vi "Autonomous Independent.vi"   [LabVIEW 2017]
doc: "This VI is called when autonomous begins, and will automatically be terminated when autonomous ends. You can carry out timed or sensor driven robot movement independently without needing to return to the caller."
uses:
  Public/Documents/Cross The Road Electronics/Phoenix-LabVIEW/Motor Controller/Controls/CTRE_Phoenix_MotorControl_ControlMode.ctl
  <vilib>/Rock Robotics/WPI/Utilities/WPI_GetSetVariantRefNum.vi
  <vilib>/Rock Robotics/Network Tables/NT Read String.vi
  <vilib>/Rock Robotics/Network Tables/NT Write Numeric Array.vi
  Public/Documents/Cross The Road Electronics/Phoenix-LabVIEW/Motor Controller/Get/CTRE_Phoenix_MotorController_GetSelectedSensorData.vi
panel:
  # "Be sure to right-click and choose Data Operations>>Make Current Value default if you want to save the array values with the VI"
types:
  T1 = typedef "CTRE_Phoenix_MotorControl_ControlMode.ctl" = u16
  T2 = typedef "WPI_JoystickDevRef.ctl" = cluster{"Device":T3}
  T3 = typedef "WPI_JoystickDeviceEnum.ctl" = enum16{"USB 0", "USB 1", "USB 2", "USB 3", "USB 4", "USB 5"}
  T4 = typedef "WPI_GyroDevRef.ctl" = cluster{"DevStatus":errorcluster, "Analog Channel":T5, "Gain (VoltsPerDegree/Second)":dbl, "Gyro Type":enum16{"Analog", "XRS450"}, "Handle":i32, "SPI Bus":T6, "Device Found":bool, "Sample Rate":dbl, "Calibrate On Open":bool, "Offset":dbl}
  T5 = typedef "FPGA_AIChannel.ctl" = enum8{"AI 0", "AI 1", "AI 2", "AI 3", "AI MXP 0", "AI MXP 1", "AI MXP 2", "AI MXP 3", "Invalid"}
  T6 = typedef "spi_bus.ctl" = enum16{"SPI On-Board, CS0", "SPI On-Board, CS1", "SPI On-Board, CS2", "SPI On-Board, CS3", "SPI MXP", "Invalid"}
  T7 = typedef "WPI_MotorControlDeviceRef.ctl" = cluster{"DeviceStatus":errorcluster, "Type":T8, "PWM":cluster{"PWM Channel":T9, "DeadBand":T10}, "CAN":cluster{"Device Number":u8, "SetOutput VI Ref":variant, "GetOutput VI Ref":variant, "Enable VI Ref":variant, "Disable VI Ref":variant, "Data":variant}, "Invert":bool, "DIO PWM":cluster{"PWM \"Enable\" Channel":T9, "DIOChannel":T11, "PWM Rate":dbl}}
  T8 = typedef "WPI_MotorControlType.ctl" = enum16{"PWM", "CAN", "DIO PWM"}
  T9 = typedef "FPGA_DIOPWMChannel.ctl" = enum8{"PWM 0", "PWM 1", "PWM 2", "PWM 3", "PWM 4", "PWM 5", "PWM 6", "PWM 7", "PWM 8", "PWM 9", "PWM MXP 0", "PWM MXP 1", "PWM MXP 2", "PWM MXP 3", "PWM MXP 4", "PWM MXP 5", "PWM MXP 6", "PWM MXP 7", "PWM MXP 8", "PWM MXP 9", "Invalid"}
  T10 = typedef "WPI_PWMDeadband.ctl" = cluster{"Name":string, "maxPositivePwm":i32, "minPositivePwm":i32, "centerPwm":i32, "maxNegativePwm":i32, "minNegativePwm":i32, "angularRange":u16}
  T11 = typedef "FPGA_DIOChannel.ctl" = enum8{"DIO 0", "DIO 1", "DIO 2", "DIO 3", "DIO 4", "DIO 5", "DIO 6", "DIO 7", "DIO 8", "DIO 9", "DIO MXP 0", "DIO MXP 1", "DIO MXP 2", "DIO MXP 3", "DIO MXP 4", "DIO MXP 5", "DIO MXP 6", "DIO MXP 7", "DIO MXP 8", "DIO MXP 9", "DIO MXP 10", "DIO MXP 11", "DIO MXP 12", "DIO MXP 13", "DIO MXP 14", "DIO MXP 15", "SPI Port CS1", "SPI Port CS2", "SPI Port CS3", "SPI Port MISO", "SPI Port MOSI", "Invalid"}
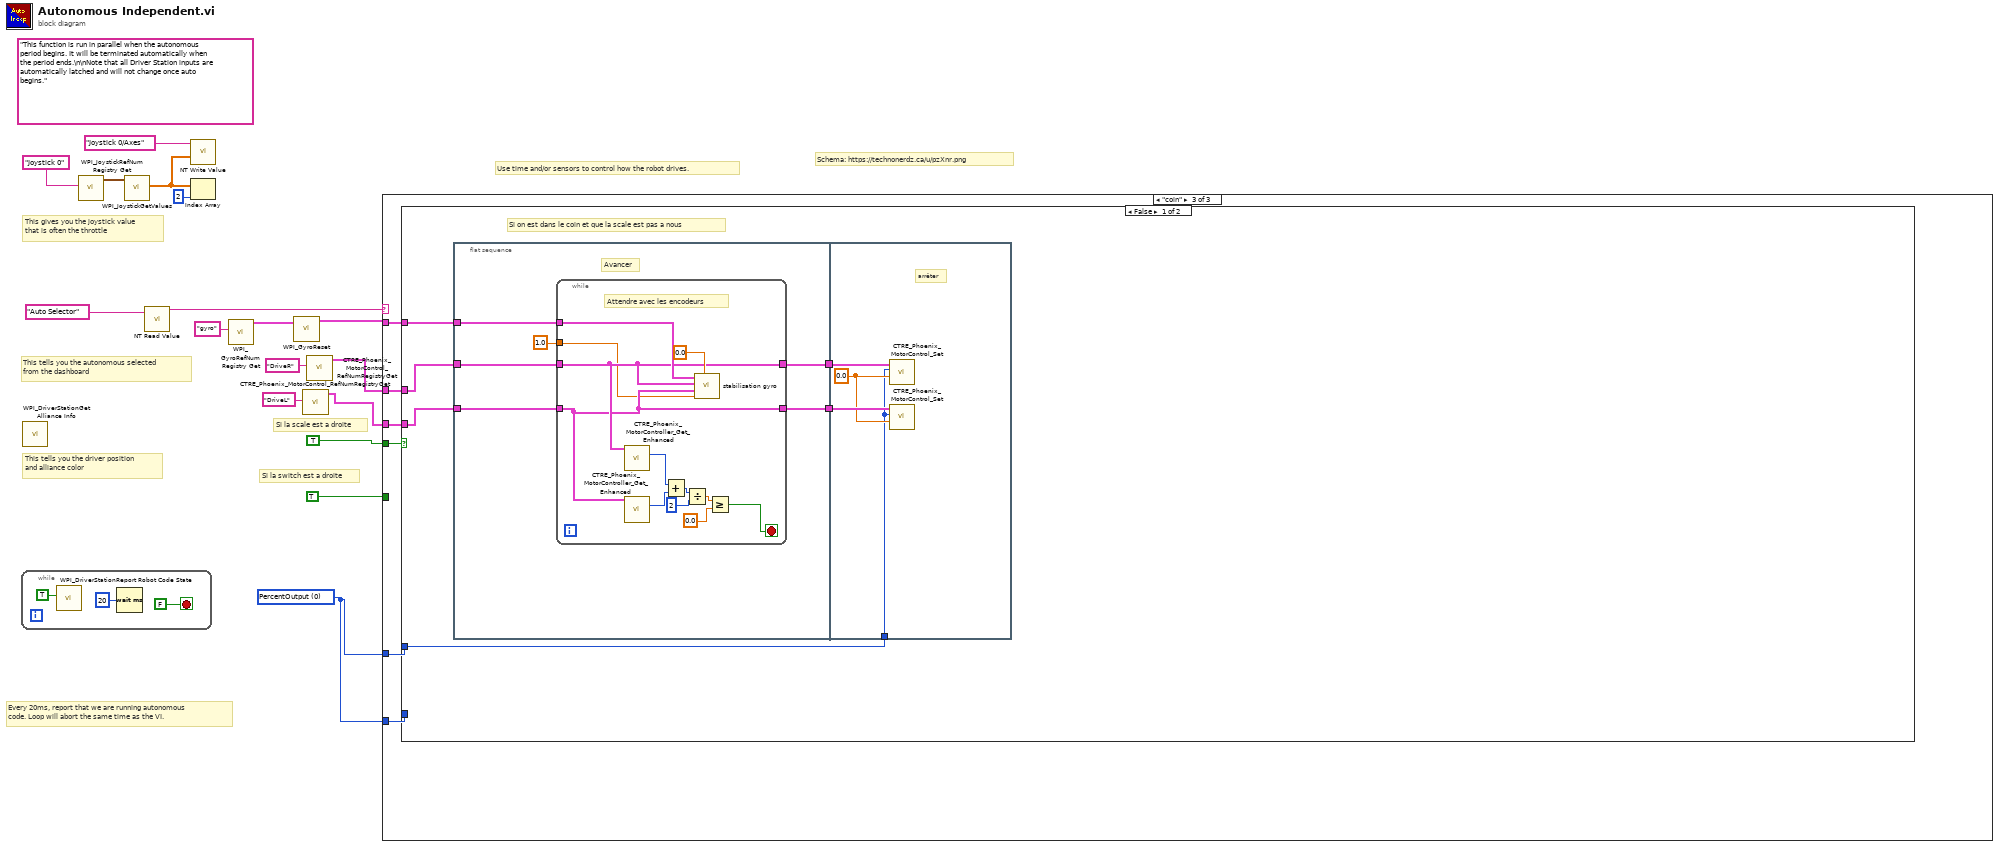
[diagram p0: block diagram]
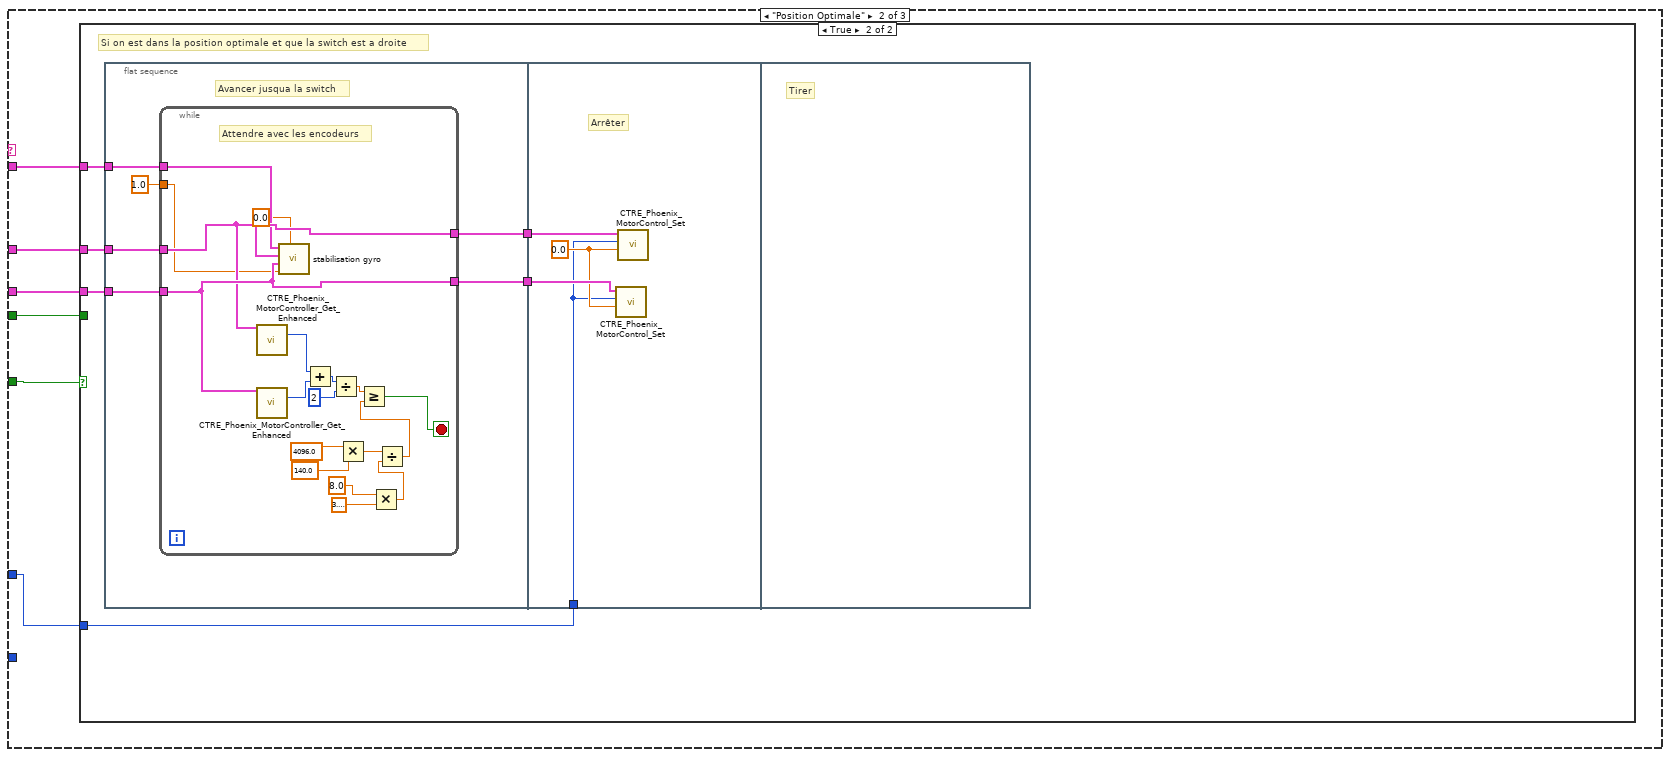
[diagram p3: hidden frame]
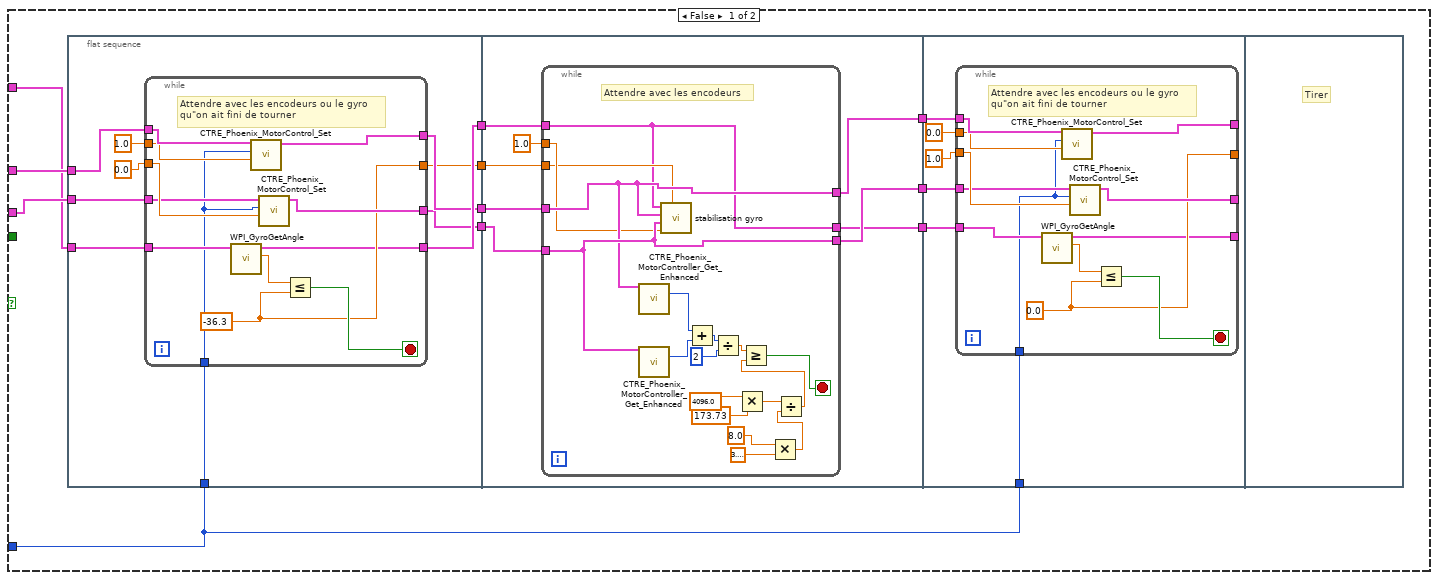
[diagram p4: hidden frame]
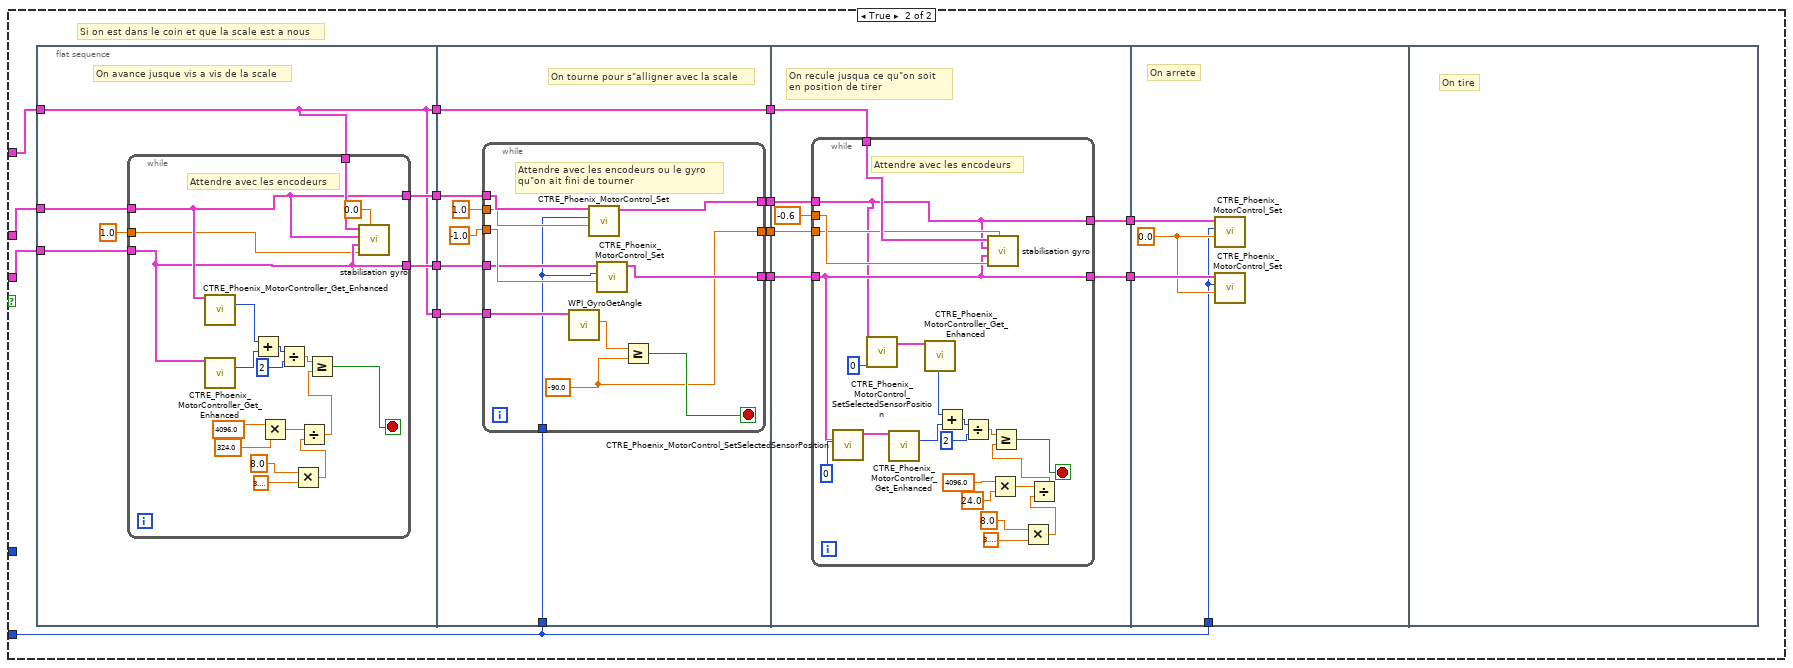
[diagram p5: hidden frame]
diagram:
  w1 = T1 0 items=["PercentOutput"=0, "Position"=1, "Velocity"=2, "Current"=3, "Follower"=5, "MotionProfile"=6, "MotionMagic"=7, "MotionMagicArc"=8, "MotionProfileArc"=10, "Disabled"=15] ("Control Mode")
  (unwired) "This function is run in parallel when the autonomous period begins. It will be terminated automatically when the period ends.\n\nNote that all Driver Station inputs are automatically latched and will not change once auto begins."
  # "Schema: https://technonerdz.ca/u/pzXnr.png"
  # "Si la switch est a droite"
  # "Si la scale est a droite"
  # "This tells you the autonomous selected\nfrom the dashboard"
  # "Every 20ms, report that we are running autonomous\ncode. Loop will abort the same time as the VI."
  # "This gives you the joystick value\nthat is often the throttle"
  # "Use time and/or sensors to control how the robot drives."
  # "This tells you the driver position\nand alliance color"
  n1 = while {
    stop <- FALSE stop-if-true
    n2 = call <vilib>:"WPI_DriverStationReport Robot Code State.vi"("Autonomous"=TRUE) -> ()  [unwired: 10 in, 1 out]
    n3 = Wait (ms)(milliseconds to wait=u32 20) -> ()  [unwired: 1 out]
  }
  n4 = call <vilib>:"WPI_DriverStationGet Alliance Info.vi"() -> ()  [unwired: 12 out]
  n5 = call <vilib>:"WPI_JoystickRefNum Registry Get.vi"("refnum name"="Joystick 0") -> ("JoystickDevRef"=w16:T2)  [unwired: 1 in, 9 out]
  n6 = call <vilib>:"WPI_JoystickGetValues.vi"("JoystickDevRef"=w16) -> ("Axes"=w12:dbl[])  [unwired: 6 in, 4 out]
  n7 = call-poly <vilib>:"NT Read Value.vi"("Name"="Auto Selector") -> ("String"=w13:string)  [unwired: 9 in, 1 out]
  n8 = call-poly <vilib>:"NT Write Value.vi"("Numeric Array"=w12, "Name"="Joystick 0/Axes") -> ()  [unwired: 9 in, 1 out]
  n9 = Index Array(array=w12, index=2) -> ()  [unwired: 1 out]
  n10 = call <vilib>:"WPI_GyroRefNum Registry Get.vi"("refnum name"="gyro") -> ("GyroDevRef"=w3:T4)  [unwired: 9 in, 1 out]
  n11 = call <vilib>:"WPI_GyroReset.vi"("GyroDevRef"=w3) -> ("GyroDevRef"=w2:T4)  [unwired: 9 in, 1 out]
  n12 = call "CTRE_Phoenix_MotorControl_RefNumRegistryGet.vi"("refnum name"="DriveL") -> ("PhoenixMotorControlDevRef"=w5:T7)  [unwired: 9 in, 1 out]
  n13 = call "CTRE_Phoenix_MotorControl_RefNumRegistryGet.vi"("refnum name"="DriveR") -> ("PhoenixMotorControlDevRef"=w6:T7)  [unwired: 9 in, 1 out]
  n14 = case shown="\"coin\"" w13 {
    tunnel: TRUE -> [_ w25 w143]
    tunnel: TRUE -> [_ w26 _]
    tunnel: w6 -> [_ w24 w142]
    tunnel: w5 -> [_ w23 w141]
    tunnel: w2 -> [_ w22 w140]
    tunnel: w1 -> [_ _ w139]
    tunnel: w1 -> [_ w21 w138]
    frame Default {
      # "You can put your main auto here, or you can right-click on the case and make any\nother frame be the default case."
      # "This is the frame that will execute if no selection is made, or if it is not recognized"
    }
    frame "Position Optimale" {
      n15 = case shown="True" w26 {
        tunnel: w25 -> [_ _]
        tunnel: w24 -> [w37 w109]
        tunnel: w23 -> [w36 w108]
        tunnel: w22 -> [w35 w105]
        tunnel: w21 -> [w27 w104]
        frame False {
          n16 = flat-sequence {
            tunnel: w37 -> [w45]
            tunnel: w36 -> [w44]
            tunnel: w35 -> [w43]
            tunnel: w27 -> [w42]
            tunnel: [w41] -> w34
            tunnel: [w40] -> w33
            tunnel: [w39] -> w32
            tunnel: [w38] -> w31
            tunnel: w34 -> [w66]
            tunnel: w33 -> [w65]
            tunnel: w32 -> [w64]
            tunnel: w31 -> [w63]
            tunnel: [w62] -> w30
            tunnel: [w61] -> w29
            tunnel: [w60] -> w28
            tunnel: w30 -> [w89]
            tunnel: w29 -> [w88]
            tunnel: w28 -> [w87]
            tunnel: w27 -> [w86]
            frame #0 {
              n17 = while {
                tunnel: 0.0 ("left") -> [w57]
                tunnel: 1.0 ("right") -> [w58]
                tunnel: w45 -> [w59]
                tunnel: w44 -> [w56]
                tunnel: [w55] -> w40
                tunnel: [w54] -> w39
                tunnel: w43 -> [w51]
                tunnel: [w50] -> w38
                tunnel: w42 -> [w49]
                tunnel: [w48] -> w41
                stop <- w52 stop-if-true
                w50 = -36.3 ("y")
                # "Attendre avec les encodeurs ou le gyro\nqu\"on ait fini de tourner"
                n18 = call <vilib>:"WPI_GyroGetAngle.vi"("GyroDevRef"=w51) -> ("Angle"=w53:dbl, "GyroDevRef"=w48:T4)  [unwired: 6 in, 3 out]
                n19 = call "CTRE_Phoenix_MotorControl_Set.vi"("Output"=w58, "Control Mode"=w49, "PhoenixMotorControlDevRef"=w59) -> ("PhoenixMotorControlDevRef"=w55:T7)  [unwired: 7 in, 1 out]
                n20 = call "CTRE_Phoenix_MotorControl_Set.vi"("Output"=w57, "Control Mode"=w49, "PhoenixMotorControlDevRef"=w56) -> ("PhoenixMotorControlDevRef"=w54:T7)  [unwired: 7 in, 1 out]
                n21 = Less Or Equal?(x=w53, y=w50) -> (x <= y?=w52:bool)
              }
            }
            frame #1 {
              n22 = while {
                tunnel: 1.0 ("right") -> [w77]
                tunnel: w65 -> [w78]
                tunnel: w64 -> [w79]
                tunnel: [w79] -> w61
                tunnel: [w78] -> w62
                tunnel: w66 -> [w75]
                tunnel: w63 -> [w76]
                tunnel: [w75] -> w60
                stop <- w80 stop-if-true
                # "Attendre avec les encodeurs"
                n23 = call-poly "CTRE_Phoenix_MotorController_Get_Enhanced.vi"("PhoenixMotorControlDevRef"=w78) -> ("Position (Raw Sensor Units)"=w85:i32)  [unwired: 11 in, 3 out]
                n24 = call-poly "CTRE_Phoenix_MotorController_Get_Enhanced.vi"("PhoenixMotorControlDevRef"=w79) -> ("Position (Raw Sensor Units)"=w84:i32)  [unwired: 11 in, 3 out]
                n25 = call "stabilisation gyro.vi"("Direction degres"=w76, "speed"=w77, "LeftMotorDevRef"=w79, "RightMotorDevRef"=w78, "gyroDevRef"=w75) -> ()  [unwired: 7 in]
                n26 = Add(x=w85, y=w84) -> (x+y=w83:i32)
                n27 = Divide(x=w83, y=2) -> (x/y=w81:dbl)
                n28 = Multiply(x=4096.0, y=173.73) -> (x*y=w70:dbl)
                n29 = Multiply(x=8.0, y=3.141592653589793) -> (x*y=w69:dbl)
                n30 = Divide(x=w70, y=w69) -> (x/y=w68:dbl)
                n31 = Greater Or Equal?(x=w81, y=w68) -> (x >= y?=w80:bool)
              }
            }
            frame #2 {
              n32 = while {
                tunnel: 1.0 ("left") -> [w101]
                tunnel: 0.0 ("right") -> [w102]
                tunnel: w89 -> [w103]
                tunnel: w88 -> [w100]
                tunnel: [w99] -> _
                tunnel: [w98] -> _
                tunnel: [w95] -> _
                tunnel: [w94] -> _
                tunnel: w87 -> [w93]
                tunnel: w86 -> [w92]
                stop <- w96 stop-if-true
                w95 = 0.0 ("y")
                # "Attendre avec les encodeurs ou le gyro\nqu\"on ait fini de tourner"
                n33 = call <vilib>:"WPI_GyroGetAngle.vi"("GyroDevRef"=w93) -> ("Angle"=w97:dbl, "GyroDevRef"=w94:T4)  [unwired: 6 in, 3 out]
                n34 = call "CTRE_Phoenix_MotorControl_Set.vi"("Output"=w102, "Control Mode"=w92, "PhoenixMotorControlDevRef"=w103) -> ("PhoenixMotorControlDevRef"=w99:T7)  [unwired: 7 in, 1 out]
                n35 = call "CTRE_Phoenix_MotorControl_Set.vi"("Output"=w101, "Control Mode"=w92, "PhoenixMotorControlDevRef"=w100) -> ("PhoenixMotorControlDevRef"=w98:T7)  [unwired: 7 in, 1 out]
                n36 = Less Or Equal?(x=w97, y=w95) -> (x <= y?=w96:bool)
              }
            }
            frame #3 {
              # "Tirer"
            }
          }
        }
        frame True {
          # "Si on est dans la position optimale et que la switch est a droite"
          n37 = flat-sequence {
            tunnel: w109 -> [w114]
            tunnel: w108 -> [w113]
            tunnel: [w112] -> w107
            tunnel: [w111] -> w106
            tunnel: w105 -> [w110]
            tunnel: w107 -> [w137]
            tunnel: w106 -> [w136]
            tunnel: w104 -> [w134]
            frame #0 {
              # "Avancer jusqua la switch"
              n38 = while {
                tunnel: 1.0 ("right") -> [w123]
                tunnel: w114 -> [w126]
                tunnel: w113 -> [w127]
                tunnel: [w127] -> w112
                tunnel: [w126] -> w111
                tunnel: w110 -> [w125]
                stop <- w128 stop-if-true
                # "Attendre avec les encodeurs"
                n39 = call-poly "CTRE_Phoenix_MotorController_Get_Enhanced.vi"("PhoenixMotorControlDevRef"=w126) -> ("Position (Raw Sensor Units)"=w133:i32)  [unwired: 11 in, 3 out]
                n40 = call-poly "CTRE_Phoenix_MotorController_Get_Enhanced.vi"("PhoenixMotorControlDevRef"=w127) -> ("Position (Raw Sensor Units)"=w132:i32)  [unwired: 11 in, 3 out]
                n41 = call "stabilisation gyro.vi"("Direction degres"=0.0, "speed"=w123, "LeftMotorDevRef"=w127, "RightMotorDevRef"=w126, "gyroDevRef"=w125) -> ()  [unwired: 7 in]
                n42 = Add(x=w133, y=w132) -> (x+y=w131:i32)
                n43 = Divide(x=w131, y=2) -> (x/y=w129:dbl)
                n44 = Multiply(x=4096.0, y=140.0) -> (x*y=w118:dbl)
                n45 = Multiply(x=8.0, y=3.141592653589793) -> (x*y=w117:dbl)
                n46 = Divide(x=w118, y=w117) -> (x/y=w116:dbl)
                n47 = Greater Or Equal?(x=w129, y=w116) -> (x >= y?=w128:bool)
              }
            }
            frame #1 {
              w135 = 0.0 ("Output")
              # "Arrêter"
              n48 = call "CTRE_Phoenix_MotorControl_Set.vi"("Output"=w135, "Control Mode"=w134, "PhoenixMotorControlDevRef"=w137) -> ()  [unwired: 7 in, 2 out]
              n49 = call "CTRE_Phoenix_MotorControl_Set.vi"("Output"=w135, "Control Mode"=w134, "PhoenixMotorControlDevRef"=w136) -> ()  [unwired: 7 in, 2 out]
            }
            frame #2 {
              # "Tirer"
            }
          }
        }
      }
    }
    frame "coin" {
      n50 = case shown="False" w143 {
        tunnel: w142 -> [w149 w185]
        tunnel: w141 -> [w148 w184]
        tunnel: w140 -> [w145 w177]
        tunnel: w139 -> [_ w172]
        tunnel: w138 -> [w144 _]
        frame False {
          # "Si on est dans le coin et que la scale est pas a nous"
          n51 = flat-sequence {
            tunnel: w149 -> [w154]
            tunnel: w148 -> [w153]
            tunnel: [w152] -> w147
            tunnel: [w151] -> w146
            tunnel: w145 -> [w150]
            tunnel: w147 -> [w171]
            tunnel: w146 -> [w170]
            tunnel: w144 -> [w168]
            frame #0 {
              # "Avancer"
              n52 = while {
                tunnel: 1.0 ("right") -> [w156]
                tunnel: w154 -> [w158]
                tunnel: w153 -> [w157]
                tunnel: [w158] -> w152
                tunnel: [w157] -> w151
                tunnel: w150 -> [w159]
                stop <- w161 stop-if-true
                # "Attendre avec les encodeurs"
                n53 = call-poly "CTRE_Phoenix_MotorController_Get_Enhanced.vi"("PhoenixMotorControlDevRef"=w158) -> ("Position (Raw Sensor Units)"=w167:i32)  [unwired: 11 in, 3 out]
                n54 = call-poly "CTRE_Phoenix_MotorController_Get_Enhanced.vi"("PhoenixMotorControlDevRef"=w157) -> ("Position (Raw Sensor Units)"=w166:i32)  [unwired: 11 in, 3 out]
                n55 = Add(x=w167, y=w166) -> (x+y=w165:i32)
                n56 = Divide(x=w165, y=2) -> (x/y=w163:dbl)
                n57 = call "stabilisation gyro.vi"("Direction degres"=0.0, "speed"=w156, "LeftMotorDevRef"=w157, "RightMotorDevRef"=w158, "gyroDevRef"=w159) -> ()  [unwired: 7 in]
                n58 = Greater Or Equal?(x=w163, y=0.0) -> (x >= y?=w161:bool)
              }
            }
            frame #1 {
              w169 = 0.0 ("Output")
              # "arrêter"
              n59 = call "CTRE_Phoenix_MotorControl_Set.vi"("Output"=w169, "Control Mode"=w168, "PhoenixMotorControlDevRef"=w171) -> ()  [unwired: 7 in, 2 out]
              n60 = call "CTRE_Phoenix_MotorControl_Set.vi"("Output"=w169, "Control Mode"=w168, "PhoenixMotorControlDevRef"=w170) -> ()  [unwired: 7 in, 2 out]
            }
          }
        }
        frame True {
          # "Si on est dans le coin et que la scale est a nous"
          n61 = flat-sequence {
            tunnel: [w188] -> w183
            tunnel: [w187] -> w182
            tunnel: [w186] -> w176
            tunnel: [w186] -> w175
            tunnel: w185 -> [w190]
            tunnel: w184 -> [w189]
            tunnel: w177 -> [w186]
            tunnel: w183 -> [w217]
            tunnel: w182 -> [w216]
            tunnel: [w215] -> w181
            tunnel: [w214] -> w180
            tunnel: w176 -> [w213]
            tunnel: w175 -> [w212]
            tunnel: [w212] -> w174
            tunnel: [w211] -> w173
            tunnel: w172 -> [w210]
            tunnel: w181 -> [w236]
            tunnel: w180 -> [w235]
            tunnel: [w234] -> w179
            tunnel: [w233] -> w178
            tunnel: w174 -> [w232]
            tunnel: w173 -> [w231]
            tunnel: w179 -> [w263]
            tunnel: w178 -> [w262]
            tunnel: w172 -> [w260]
            frame #0 {
              # "On avance jusque vis a vis de la scale"
              n62 = while {
                tunnel: 1.0 ("right") -> [w200]
                tunnel: w190 -> [w202]
                tunnel: w189 -> [w201]
                tunnel: [w202] -> w188
                tunnel: [w201] -> w187
                tunnel: w186 -> [w203]
                stop <- w204 stop-if-true
                # "Attendre avec les encodeurs"
                n63 = call-poly "CTRE_Phoenix_MotorController_Get_Enhanced.vi"("PhoenixMotorControlDevRef"=w202) -> ("Position (Raw Sensor Units)"=w209:i32)  [unwired: 11 in, 3 out]
                n64 = call-poly "CTRE_Phoenix_MotorController_Get_Enhanced.vi"("PhoenixMotorControlDevRef"=w201) -> ("Position (Raw Sensor Units)"=w208:i32)  [unwired: 11 in, 3 out]
                n65 = Add(x=w209, y=w208) -> (x+y=w207:i32)
                n66 = Multiply(x=4096.0, y=324.0) -> (x*y=w194:dbl)
                n67 = Divide(x=w207, y=2) -> (x/y=w205:dbl)
                n68 = Multiply(x=8.0, y=3.141592653589793) -> (x*y=w193:dbl)
                n69 = Divide(x=w194, y=w193) -> (x/y=w192:dbl)
                n70 = Greater Or Equal?(x=w205, y=w192) -> (x >= y?=w204:bool)
                n71 = call "stabilisation gyro.vi"("Direction degres"=0.0, "speed"=w200, "LeftMotorDevRef"=w201, "RightMotorDevRef"=w202, "gyroDevRef"=w203) -> ()  [unwired: 7 in]
              }
            }
            frame #1 {
              # "On tourne pour s\"alligner avec la scale"
              n72 = while {
                tunnel: -1.0 ("left") -> [w228]
                tunnel: 1.0 ("right") -> [w229]
                tunnel: w217 -> [w230]
                tunnel: w216 -> [w227]
                tunnel: [w226] -> w215
                tunnel: [w225] -> w214
                tunnel: w213 -> [w222]
                tunnel: [w221] -> w211
                tunnel: w210 -> [w220]
                stop <- w223 stop-if-true
                w221 = -90.0 ("y")
                # "Attendre avec les encodeurs ou le gyro\nqu\"on ait fini de tourner"
                n73 = call <vilib>:"WPI_GyroGetAngle.vi"("GyroDevRef"=w222) -> ("Angle"=w224:dbl)  [unwired: 6 in, 4 out]
                n74 = call "CTRE_Phoenix_MotorControl_Set.vi"("Output"=w229, "Control Mode"=w220, "PhoenixMotorControlDevRef"=w230) -> ("PhoenixMotorControlDevRef"=w226:T7)  [unwired: 7 in, 1 out]
                n75 = call "CTRE_Phoenix_MotorControl_Set.vi"("Output"=w228, "Control Mode"=w220, "PhoenixMotorControlDevRef"=w227) -> ("PhoenixMotorControlDevRef"=w225:T7)  [unwired: 7 in, 1 out]
                n76 = Greater Or Equal?(x=w224, y=w221) -> (x >= y?=w223:bool)
              }
            }
            frame #2 {
              # "On recule jusqua ce qu\"on soit\nen position de tirer"
              n77 = while {
                tunnel: -0.6 ("right") -> [w253]
                tunnel: w236 -> [w247]
                tunnel: w235 -> [w249]
                tunnel: [w247] -> w234
                tunnel: [w249] -> w233
                tunnel: w232 -> [w252]
                tunnel: w231 -> [w251]
                stop <- w254 stop-if-true
                # "Attendre avec les encodeurs"
                n78 = call "CTRE_Phoenix_MotorControl_SetSelectedSensorPosition.vi"("New Sensor Position"=0, "PhoenixMotorControlDevRef"=w249) -> ("PhoenixMotorControlDevRef"=w248:T7)  [unwired: 8 in, 1 out]
                n79 = call "CTRE_Phoenix_MotorControl_SetSelectedSensorPosition.vi"("New Sensor Position"=0, "PhoenixMotorControlDevRef"=w247) -> ("PhoenixMotorControlDevRef"=w245:T7)  [unwired: 8 in, 1 out]
                n80 = call-poly "CTRE_Phoenix_MotorController_Get_Enhanced.vi"("PhoenixMotorControlDevRef"=w248) -> ("Position (Raw Sensor Units)"=w258:i32)  [unwired: 11 in, 3 out]
                n81 = call-poly "CTRE_Phoenix_MotorController_Get_Enhanced.vi"("PhoenixMotorControlDevRef"=w245) -> ("Position (Raw Sensor Units)"=w259:i32)  [unwired: 11 in, 3 out]
                n82 = Add(x=w259, y=w258) -> (x+y=w257:i32)
                n83 = Divide(x=w257, y=2) -> (x/y=w255:dbl)
                n84 = call "stabilisation gyro.vi"("Direction degres"=w251, "speed"=w253, "LeftMotorDevRef"=w249, "RightMotorDevRef"=w247, "gyroDevRef"=w252) -> ()  [unwired: 7 in]
                n85 = Multiply(x=4096.0, y=24.0) -> (x*y=w243:dbl)
                n86 = Multiply(x=8.0, y=3.141592653589793) -> (x*y=w244:dbl)
                n87 = Divide(x=w243, y=w244) -> (x/y=w238:dbl)
                n88 = Greater Or Equal?(x=w255, y=w238) -> (x >= y?=w254:bool)
              }
            }
            frame #3 {
              w261 = 0.0 ("Output")
              # "On arrete"
              n89 = call "CTRE_Phoenix_MotorControl_Set.vi"("Output"=w261, "Control Mode"=w260, "PhoenixMotorControlDevRef"=w263) -> ()  [unwired: 7 in, 2 out]
              n90 = call "CTRE_Phoenix_MotorControl_Set.vi"("Output"=w261, "Control Mode"=w260, "PhoenixMotorControlDevRef"=w262) -> ()  [unwired: 7 in, 2 out]
            }
            frame #4 {
              # "On tire"
            }
          }
        }
      }
    }
  }
